vi "Init Default Views.vi"(6 "MainPane Actor":refnum<class "MainView.lvclass">, 8 "error in (no error)":errorcluster, 9 "CharmView Actor":refnum<class "CharmView.lvclass">, 10 "AppBarView Actor":refnum<class "AppBarView.lvclass">, 11 "MainController in":refnum<class "MainController.lvclass">) -> (0 "error out":errorcluster, 3 "MainController out":refnum<class "MainController.lvclass">)   [LabVIEW 2012, in "Win8uiFramework.lvlib" / "MainController.lvclass"]
doc: "Override this VI to provide default Actors for each SubView."
uses:
  MainController.lvclass
  MainView.lvclass
  CharmView.lvclass
  AppBarView.lvclass
  MainController.lvclass/MainController.ctl
  Insert Into SubPanel Msg.lvclass/Insert Into SubPanel Msg.ctl
  <vilib>/ActorFramework/Message Enqueuer/Message Enqueuer.lvclass/Message Enqueuer.ctl
  Write Default AppBar Actor.vi
  Write Default Charm Actor.vi
  Write Default MainPane Actor.vi
  Read MainPane Enqueuer.vi
  Read Active SubPanel.vi
  <vilib>/ActorFramework/Message Enqueuer/Enqueue.vi
  <vilib>/ActorFramework/Message Priority Queue/Priority Enqueue.vi
  <vilib>/ActorFramework/Message Enqueuer/Message Enqueuer.lvclass
  Insert Into SubPanel Msg.lvclass
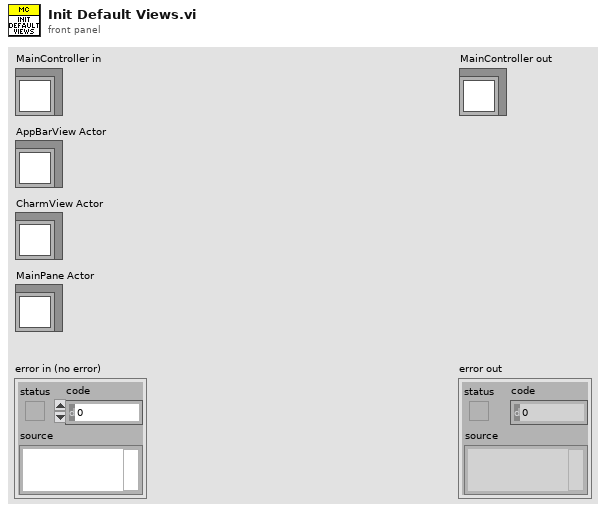
[diagram p1: front panel]
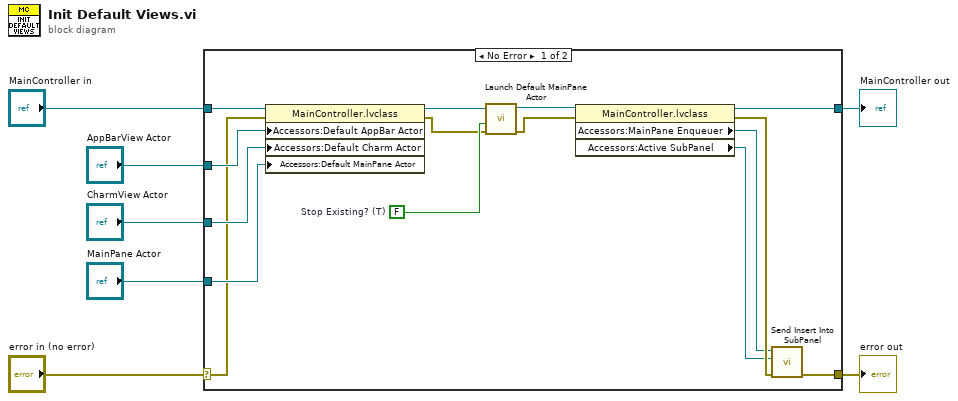
[diagram p0: block diagram]
diagram:
  n1 = case shown="No Error" "error in (no error)" {
    selector: "error in (no error)" -> [w15 w24]
    tunnel: [w19 w24] -> w6
    tunnel: [w22 w23] -> w4
    tunnel: "MainController in" -> [w21 w23]
    tunnel: "CharmView Actor" -> [w17 _]
    tunnel: "AppBarView Actor" -> [w18 _]
    tunnel: "MainPane Actor" -> [w16 _]
    frame No Error {
      w12 = FALSE  # Stop Existing? (T)
      n2 = property class="MainController.lvclass"(reference=w21, error in=w15, "Accessors:Default AppBar Actor"=w18, "Accessors:Default Charm Actor"=w17, "Accessors:Default MainPane Actor"=w16) -> (reference out=w10:refnum<class "MainController.lvclass">, error out=w11:errorcluster)
      n3 = call-dynamic "Launch Default MainPane Actor.vi"("error in (no error)"=w11, "Stop Existing? (T)"=w12, "MainController in"=w10) -> ("error out"=w9:errorcluster, "MainController out"=w8:refnum<class "MainController.lvclass">)  [unwired: 6 in, 1 out]
      n4 = property class="MainController.lvclass"(reference=w8, error in=w9) -> (reference out=w22:refnum<class "MainController.lvclass">, error out=w20:errorcluster, "Accessors:MainPane Enqueuer"=w14:refnum<class "Message Enqueuer.lvclass">, "Accessors:Active SubPanel"=w13:refnum<vi>)
      n5 = call "Send Insert Into SubPanel.vi"("error in (no error)"=w20, "SubPanel Ref"=w13, "Message Enqueuer"=w14) -> ("error out"=w19:errorcluster)  [unwired: 7 in, 1 out]
    }
    frame Error {
    }
  }
  "error out" <- w6
  "MainController out" <- w4
